vi "PDC_GetShutterSpeedFps.vi"(8 "error in (no error)":errorcluster, 10 "ChildNo":u32, 11 "DeviceNo":u32) -> (0 "error out":errorcluster, 2 "Fps":u32, 3 "ReturnValue":u32, 4 "ErrorCode":u32)   [LabVIEW 2015]
doc: "This VI retrieves the shutter speed, in fractions of a second, of the specified child device."
uses:
  PDCLIB.dll
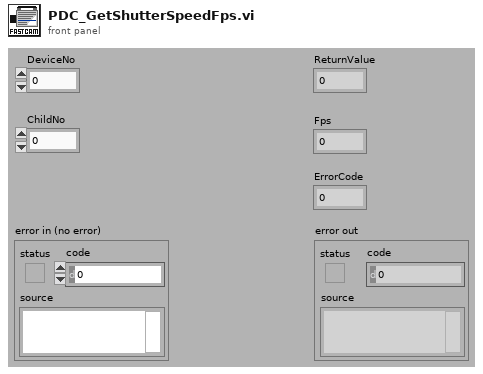
[diagram p1: front panel]
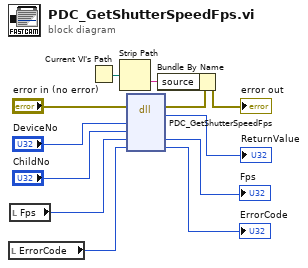
[diagram p0: block diagram]
diagram:
  n1 = local read "ErrorCode"() -> (w9:u32)
  n2 = local read "Fps"() -> (w6:u32)
  n3 = Current VI's Path() -> (path=w3:path)
  n4 = Strip Path(path=w3) -> (name=w4:string)  [unwired: 1 out]
  n5 = dll-call lib="PDCLIB.dll" fn="PDC_GetShutterSpeedFps"(error in="error in (no error)", "nDeviceNo"="DeviceNo", "nChildNo"="ChildNo", "pFps"=w6, "pErrorCode"=w9) -> (error out=w2:errorcluster, "return type"=→"ReturnValue":u32, "pFps"=→"Fps":u32, "pErrorCode"=→"ErrorCode":u32)  [unwired: 4 in, 1 out]
  n6 = Bundle By Name(cluster=w2, "source"=w4) -> (→"error out":errorcluster)
